vi "仪器电源管理.vi"() -> ()   [LabVIEW 2016, in "环境动力监测库.lvlib" / "V电源管理库.lvlib"]
uses:
  <vilib>/Utility/miscctls.llb/LVPointTypeDef.ctl
  <vilib>/ptbypt/NI_PtbyPt.lvlib
panel:
  out "R115":i16 caption="灯带关闭时间"
  out "R114":i16 caption="灯带开启时间"
  in  "照明":bool
  in  "侧边灯带":bool
  in  "电源控制":T1
  in  "主屏看门狗启用":u16(ring) caption="主屏看门狗启用：" items=["关闭", "打开"]
  in  "主屏看门狗设置":i16 caption="主屏看门狗设置："
  out "主屏看门狗计时":i16 caption="主屏看门狗计时："
  # "仪器电源管理"
  # "H"
  # "H"
  # "s"
  # "s"
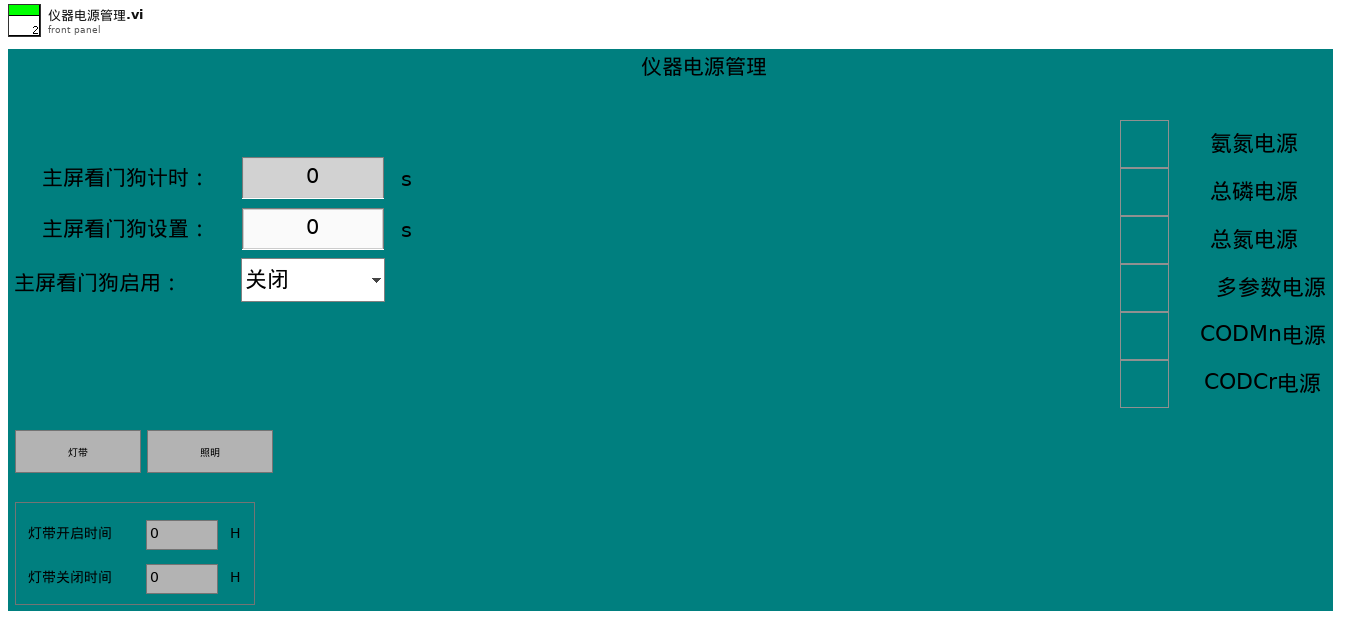
[diagram p1: front panel]
types:
  T1 = cluster{"氨氮电源":bool, "总磷电源":bool, "总氮电源":bool, "多参数电源":bool, "CODMn电源":bool, "CODCr电源":bool}
  T2 = typedef "LVPointTypeDef.ctl" = cluster{"Horizontal":i16, "Vertical":i16}
  T3 = cluster{"状态":cluster{"R0":i16, "R1":i16, "R2":i16, "R3":i16, "R4":i16, "R5":i16, "R6":i16, "R7":i16, "R8":i16, "R9":i16, "R10":i16, "R11":i16, "R12":i16, "R13":i16, "R14":i16, "R15":i16, "R16":i16, "R17":i16, "R18":i16, "R19":i16, "R20":i16, "R21":i16, "R22":i16, "R23":i16, "R24":i16, "R25":i16, "R26":i16, "R27":i16, "R28":i16, "R29":i16, "R30":i16, "R31":i16, "R32":i16, "R33":i16, "R34":i16, "R35":i16, "R36":i16, "R37":i16, "R38":i16, "R39":i16, "R40":i16, "R41":i16, "R42":i16, "R43":i16, "R44":i16, "R45":i16, "R46":i16, "R47":i16, "R48":i16, "R49":i16, "R50":i16, "R51":i16, "R52":i16, "R53":i16, "R54":i16, "R55":i16, "R56":i16, "R57":i16, "R58":i16, "R59":i16, "R60":i16, "R61":i16, "R62":i16, "R63":i16, "R64":i16, "R65":i16, "R66":i16, "R67":i16, "R68":i16, "R69":i16}, "输入状态":bool[], "输出状态":bool[], "报警簇":bool[], "参数设置":cluster{"R100":i16, "R101":i16, "R102":i16, "R103":i16, "R104":i16, "R105":i16, "R106":i16, "R107":i16, "R108":i16, "R109":i16, "R110":i16, "R111":i16, "R112":i16, "R113":i16, "R114":i16, "R115":i16, "R116":i16, "R117":i16, "R118":i16, "R119":i16, "R120":i16, "R121":i16, "R122":i16, "R123":i16, "R124":i16}, "转换值":cluster{"AD0":sgl, "AD1":sgl, "AD2":sgl, "AD3":sgl, "AD4":sgl, "AD5":sgl}, "看门狗启用":bool, "氨氮模块名称":string, "总磷模块名称":string}
  T4 = cluster{"采配水启用":bool, "CODMn启用":bool, "CODcr启用":bool, "氨氮启用":bool, "总磷启用":bool, "质控单元启用":bool, "流量计启用":bool, "电源管理启用":bool, "其他启用":bool, "多参数启用":bool, "超标留样启用":bool, "总氮启用":bool, "运行模式":enum16{"维护模式", "常规模式", "应急模式", "质控模式"}}
  T5 = cluster{"R100":i16, "R101":i16, "R102":i16, "R103":i16, "R104":i16, "R105":i16, "R106":i16, "R107":i16, "R108":i16, "R109":i16, "R110":i16, "R111":i16, "R112":i16, "R113":i16, "R114":i16, "R115":i16, "R116":i16, "R117":i16, "R118":i16, "R119":i16, "R120":i16, "R121":i16, "R122":i16, "R123":i16, "R124":i16}
  T6 = cluster{"R0":i16, "R1":i16, "R2":i16, "R3":i16, "R4":i16, "R5":i16, "R6":i16, "R7":i16, "R8":i16, "R9":i16, "R10":i16, "R11":i16, "R12":i16, "R13":i16, "R14":i16, "R15":i16, "R16":i16, "R17":i16, "R18":i16, "R19":i16, "R20":i16, "R21":i16, "R22":i16, "R23":i16, "R24":i16, "R25":i16, "R26":i16, "R27":i16, "R28":i16, "R29":i16, "R30":i16, "R31":i16, "R32":i16, "R33":i16, "R34":i16, "R35":i16, "R36":i16, "R37":i16, "R38":i16, "R39":i16, "R40":i16, "R41":i16, "R42":i16, "R43":i16, "R44":i16, "R45":i16, "R46":i16, "R47":i16, "R48":i16, "R49":i16, "R50":i16, "R51":i16, "R52":i16, "R53":i16, "R54":i16, "R55":i16, "R56":i16, "R57":i16, "R58":i16, "R59":i16, "R60":i16, "R61":i16, "R62":i16, "R63":i16, "R64":i16, "R65":i16, "R66":i16, "R67":i16, "R68":i16, "R69":i16}
  T7 = cluster{"命令":string, "data":cluster{"starting address":u16, "coil values":bool[]}}
  T8 = cluster{"命令":string, "数据":cluster{"starting address":u16, "holding register values":u16[]}}
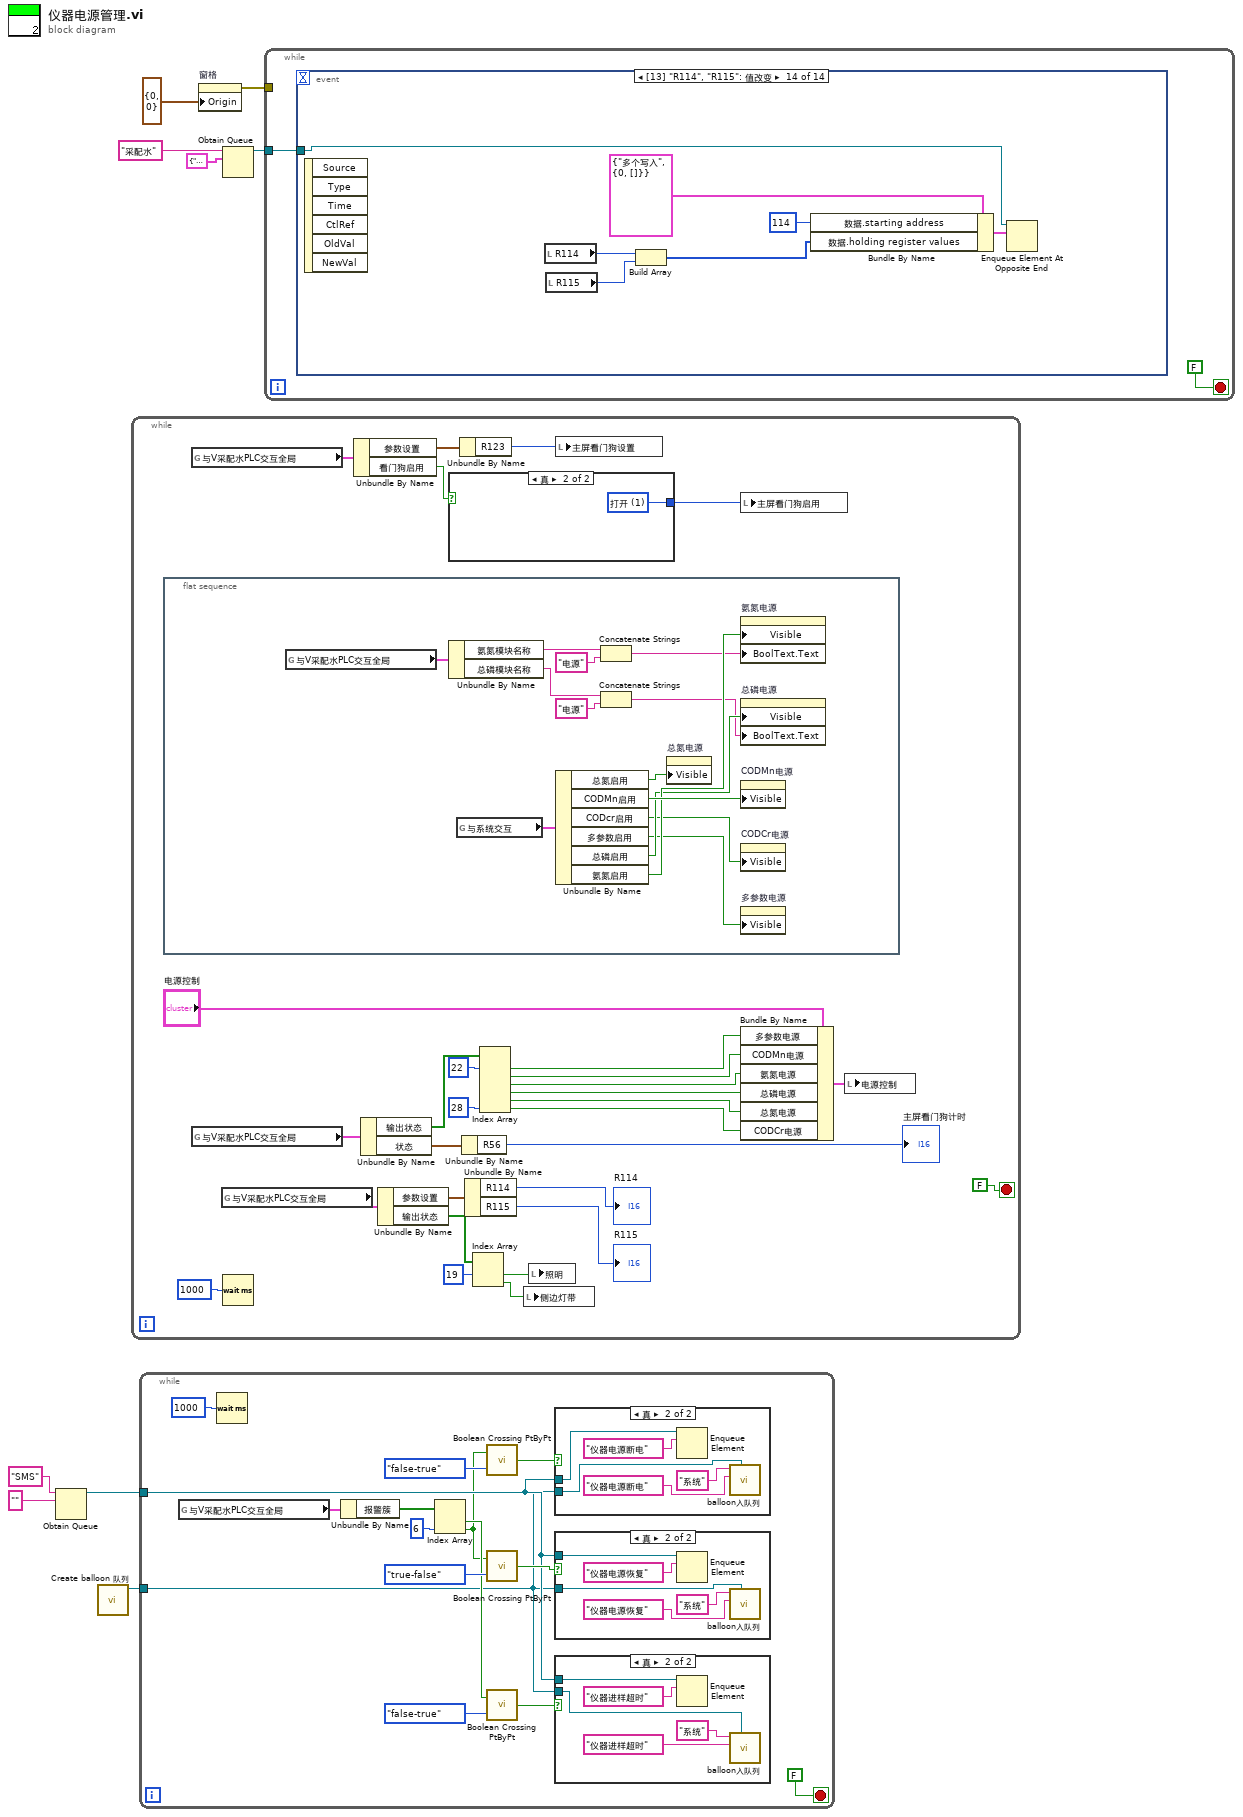
[diagram p0: block diagram]
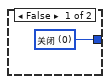
[diagram p5: hidden frame]
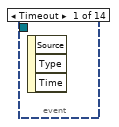
[diagram p6: hidden frame]
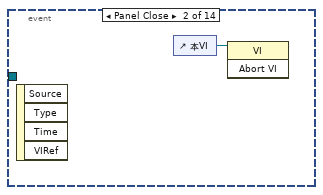
[diagram p7: hidden frame]
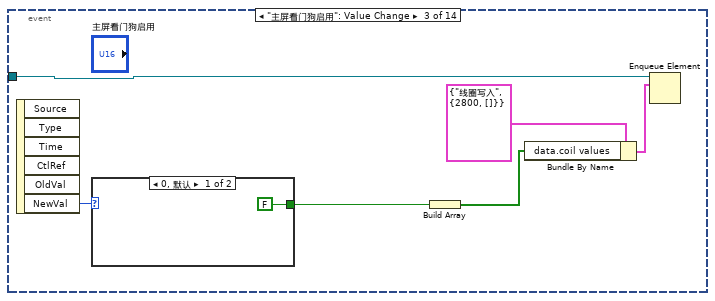
[diagram p8: hidden frame]
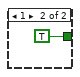
[diagram p9: hidden frame]
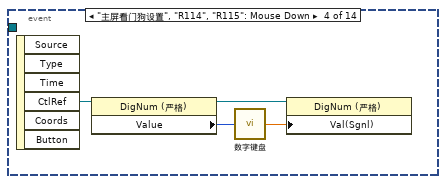
[diagram p10: hidden frame]
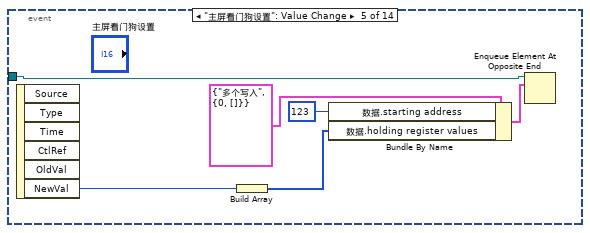
[diagram p11: hidden frame]
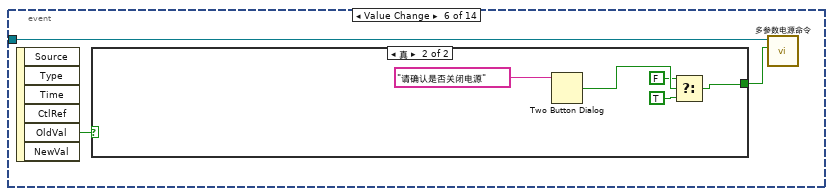
[diagram p12: hidden frame]
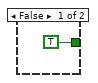
[diagram p13: hidden frame]
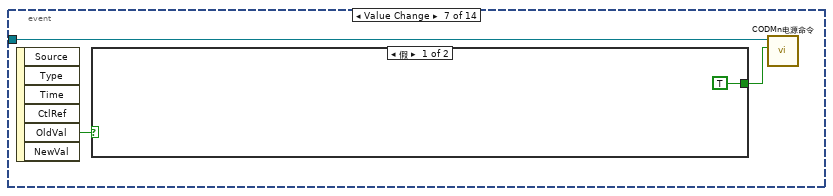
[diagram p14: hidden frame]
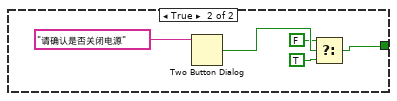
[diagram p15: hidden frame]
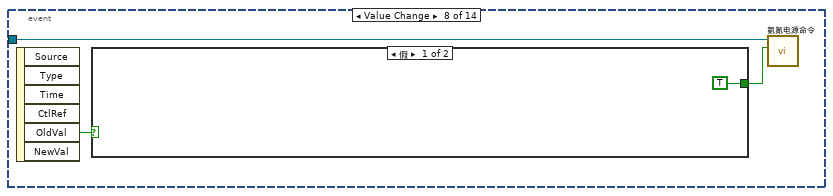
[diagram p16: hidden frame]
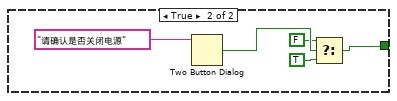
[diagram p17: hidden frame]
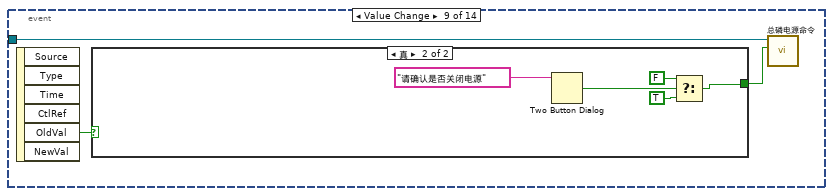
[diagram p18: hidden frame]
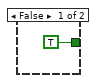
[diagram p19: hidden frame]
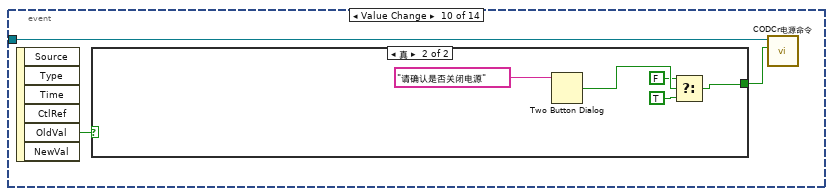
[diagram p20: hidden frame]
diagram:
  n1 = Obtain Queue(name (unnamed)="SMS" ("名称（未命名）"), element data type="" ("名称（未命名）")) -> (queue out=w2:refnum<queue>)  [unwired: 3 in, 2 out]
  n2 = call "Create balloon 队列.vi"() -> ("队列输出"=w1:refnum<queue>)  [unwired: 11 in]
  n3 = while {
    stop <- FALSE stop-if-true
    n4 = flat-sequence {
      frame #0 {
        n5 = global read "外部交互全局变量.vi" "与V采配水PLC交互全局"() -> (w46:T3)
        n6 = Unbundle By Name(w46) -> ("氨氮模块名称"=w45:string, "总磷模块名称"=w42:string)
        n7 = global read "外部交互全局变量.vi" "与系统交互"() -> (w54:T4)
        n8 = Unbundle By Name(w54) -> ("总氮启用"=w53:bool, "CODMn启用"=w52:bool, "CODcr启用"=w48:bool, "多参数启用"=w49:bool, "总磷启用"=w50:bool, "氨氮启用"=w51:bool)
        n9 = Concatenate Strings(w45, "电源" ("字符串")) -> (w44:string)
        n10 = Concatenate Strings(w42, "电源" ("字符串")) -> (w41:string)
        n11 = property on="总氮电源" class="Bool (严格)"("Visible"=w53) -> ()  [unwired: 2 in, 2 out]
        n12 = property on="氨氮电源" class="Bool (严格)"("Visible"=w51, "BoolText.Text"=w44) -> ()  [unwired: 2 in, 2 out]
        n13 = property on="总磷电源" class="Bool (严格)"("Visible"=w50, "BoolText.Text"=w41) -> ()  [unwired: 2 in, 2 out]
        n14 = property on="CODMn电源" class="Bool (严格)"("Visible"=w52) -> ()  [unwired: 2 in, 2 out]
        n15 = property on="CODCr电源" class="Bool (严格)"("Visible"=w48) -> ()  [unwired: 2 in, 2 out]
        n16 = property on="多参数电源" class="Bool (严格)"("Visible"=w49) -> ()  [unwired: 2 in, 2 out]
      }
    }
    n17 = global read "外部交互全局变量.vi" "与V采配水PLC交互全局"() -> (w25:T3)
    n18 = global read "外部交互全局变量.vi" "与V采配水PLC交互全局"() -> (w23:T3)
    n19 = global read "外部交互全局变量.vi" "与V采配水PLC交互全局"() -> (w17:T3)
    n20 = Wait (ms)(milliseconds to wait=u32 1000 ("等待时间（毫秒）")) -> ()  [unwired: 1 out]
    n21 = Unbundle By Name(w25) -> ("参数设置"=w24:T5, "看门狗启用"=w19:bool)
    n22 = Unbundle By Name(w23) -> ("输出状态"=w21:bool[], "状态"=w22:T6)
    n23 = Unbundle By Name(w17) -> ("参数设置"=w16:T5, "输出状态"=w12:bool[])
    n24 = case shown="真" w19 {
      tunnel: [w39 w40] -> w18
      frame False {
        w39 = u16 0 items=["关闭", "打开"] ("主屏看门狗启用")
      }
      frame True {
        w40 = u16 1 items=["关闭", "打开"] ("主屏看门狗启用")
      }
    }
    n25 = Unbundle By Name(w24) -> ("R123"=w35:i16)
    n26 = Unbundle By Name(w22) -> ("R56"=→"主屏看门狗计时":i16)
    n27 = Unbundle By Name(w16) -> ("R114"=→"R114":i16, "R115"=→"R115":i16)
    n28 = Index Array(array=w12, index #1=19 ("索引")) -> (element #1=w11:bool, element #2=w10:bool)  [unwired: 1 in]
    n29 = Index Array(array=w21, index #1=22 ("索引"), index #6=28 ("索引")) -> (element #1=w32:bool, element #2=w31:bool, element #3=w30:bool, element #4=w29:bool, element #5=w28:bool, element #6=w27:bool)  [unwired: 4 in]
    n30 = local write "侧边灯带"(w10) -> ()
    n31 = local write "照明"(w11) -> ()
    n32 = local write "主屏看门狗设置"(w35) -> ()
    n33 = local write "主屏看门狗启用"(w18) -> ()
    n34 = Bundle By Name(cluster="电源控制", "多参数电源"=w32, "CODMn电源"=w31, "氨氮电源"=w30, "总磷电源"=w29, "总氮电源"=w28, "CODCr电源"=w27) -> (w26:T1)
    n35 = local write "电源控制"(w26) -> ()
  }
  n36 = while {
    tunnel: w2 -> [w63]
    tunnel: w1 -> [w57]
    stop <- FALSE stop-if-true
    n37 = global read "外部交互全局变量.vi" "与V采配水PLC交互全局"() -> (w56:T3)
    n38 = Wait (ms)(milliseconds to wait=u32 1000 ("等待时间（毫秒）")) -> ()  [unwired: 1 out]
    n39 = Unbundle By Name(w56) -> ("报警簇"=w55:bool[])
    n40 = Index Array(array=w55, index #2=6 ("索引")) -> (element #1=w60:bool, element #2=w58:bool)  [unwired: 1 in]
    n41 = call <vilib>:"Boolean Crossing PtByPt.vi"("direction"=enum16{"either", "false-true", "true-false"}."false-true", "input"=w58) -> ("crossing"=w66:bool)  [unwired: 1 in]
    n42 = call <vilib>:"Boolean Crossing PtByPt.vi"("direction"=enum16{"either", "false-true", "true-false"}."true-false", "input"=w58) -> ("crossing"=w64:bool)  [unwired: 1 in]
    n43 = call <vilib>:"Boolean Crossing PtByPt.vi"("direction"=enum16{"either", "false-true", "true-false"}."false-true", "input"=w60) -> ("crossing"=w61:bool)  [unwired: 1 in]
    n44 = case shown="真" w66 {
      tunnel: w63 -> [_ w84]
      tunnel: w57 -> [_ w82]
      frame False {
      }
      frame True {
        n45 = Enqueue Element(queue=w84, element="仪器电源断电" ("元素")) -> ()  [unwired: 2 in, 3 out]
        n46 = call "balloon入队列.vi"("队列"=w82, "故障信息"="仪器电源断电" ("元素"), "参数名称"="系统") -> ()  [unwired: 8 in, 1 out]
      }
    }
    n47 = case shown="真" w64 {
      tunnel: w63 -> [_ w77]
      tunnel: w57 -> [_ w76]
      frame False {
      }
      frame True {
        n48 = Enqueue Element(queue=w77, element="仪器电源恢复" ("元素")) -> ()  [unwired: 2 in, 3 out]
        n49 = call "balloon入队列.vi"("队列"=w76, "故障信息"="仪器电源恢复" ("元素"), "参数名称"="系统") -> ()  [unwired: 8 in, 1 out]
      }
    }
    n50 = case shown="真" w61 {
      tunnel: w63 -> [_ w74]
      tunnel: w57 -> [_ w72]
      frame False {
      }
      frame True {
        n51 = Enqueue Element(queue=w74, element="仪器进样超时" ("元素")) -> ()  [unwired: 2 in, 3 out]
        n52 = call "balloon入队列.vi"("队列"=w72, "故障信息"="仪器进样超时" ("元素"), "参数名称"="系统") -> ()  [unwired: 8 in, 1 out]
      }
    }
  }
  n53 = property on="窗格" class="Pane"("Origin"=T2 {"Horizontal"=0, "Vertical"=0} ("原点")) -> (error out=w6:errorcluster)  [unwired: 2 in, 1 out]
  n54 = Obtain Queue(name (unnamed)="采配水" ("名称（未命名）"), element data type=cluster{"命令":string, "数据":variant} {"命令"="", "数据"=variant}) -> (queue out=w5:refnum<queue>)  [unwired: 3 in, 2 out]
  n55 = while {
    tunnel: w5 -> [w86]
    tunnel: w6 -> [_]
    stop <- FALSE stop-if-true
    n56 = event shown="[13] \"R114\", \"R115\": 值改变" {
      selector: _ -> [_ _ _ _ _ _ _ _ _ _ _ _ _ _]
      dyn-events: _ -> [_ _ _ _ _ _ _ _ _ _ _ _ _ _]
      timeout: _ -> [_ _ _ _ _ _ _ _ _ _ _ _ _ _]
      tunnel: w86 -> [_ _ w90 _ w102 w108 w117 w126 w135 w144 w153 w161 w166 w172]
      event Timeout {
        n57 = event-data() -> ()  [unwired: 1 in, 3 out]
      }
      event Panel Close {
        n58 = event-data() -> ()  [unwired: 1 in, 4 out]
        n59 = control-ref of="本VI"() -> (w87:refnum<vi>)
        n60 = invoke class="VI" method="Abort VI"(reference=w87) -> ()  [unwired: 2 in, 3 out]
      }
      event "主屏看门狗启用": Value Change {
        n61 = event-data() -> ("NewVal"=w89:u16)  [unwired: 1 in, 5 out]
        n62 = case shown="0, 默认" w89 {
          tunnel: [FALSE TRUE] -> w88
          frame 0, Default {
          }
          frame 1 {
          }
        }
        n63 = Build Array(w88) -> (w91:bool[])
        n64 = Bundle By Name(cluster=T7 {"命令"="线圈写入", "data"={"starting address"=2800, "coil values"=[]}} ("元素"), "data.coil values"=w91) -> (w92:T7)
        n65 = Enqueue Element(queue=w90, element=w92) -> ()  [unwired: 2 in, 3 out]
      }
      event "主屏看门狗设置", "R114", "R115": Mouse Down {
        n66 = event-data() -> ("CtlRef"=w96:refnum<vi>)  [unwired: 1 in, 5 out]
        n67 = property class="DigNum (严格)"(reference=w96) -> (reference out=w98:refnum<vi>, "Value"=w99:i16)  [unwired: 1 in, 1 out]
        n68 = call "数字键盘.vi"("OldNumber"=w99) -> ("NewNumber"=w97:sgl)
        n69 = property class="DigNum (严格)"(reference=w98, "Val(Sgnl)"=w97) -> ()  [unwired: 1 in, 2 out]
      }
      event "主屏看门狗设置": Value Change {
        n70 = event-data() -> ("NewVal"=w100:i16)  [unwired: 1 in, 5 out]
        n71 = Build Array(w100) -> (w101:i16[])
        n72 = Bundle By Name(cluster=T8 {"命令"="多个写入", "数据"={"starting address"=0, "holding register values"=[]}} ("元素"), "数据.starting address"=u16 123, "数据.holding register values"=w101) -> (w103:T8)
        n73 = Enqueue Element At Opposite End(queue=w102, element=w103) -> ()  [unwired: 2 in, 3 out]
      }
      event "电源控制.多参数电源": Value Change {
        n74 = event-data() -> ("OldVal"=w107:bool)  [unwired: 1 in, 5 out]
        n75 = case shown="真" w107 {
          tunnel: [TRUE ("T button?") w110] -> w106
          frame False {
          }
          frame True {
            n76 = Two Button Dialog(message="请确认是否关闭电源" ("消息")) -> (T button?=w113:bool)  [unwired: 2 in]
            n77 = Select(t=FALSE, s=w113, f=TRUE ("T button?")) -> (s? t:f=w110:bool)
          }
        }
        n78 = call "多参数电源命令.vi"("通电/断电"=w106, "队列"=w108) -> ()  [unwired: 9 in, 1 out]
      }
      event "电源控制.CODMn电源": Value Change {
        n79 = event-data() -> ("OldVal"=w116:bool)  [unwired: 1 in, 5 out]
        n80 = case shown="假" w116 {
          tunnel: [TRUE ("T button?") w119] -> w115
          frame False {
          }
          frame True {
            n81 = Two Button Dialog(message="请确认是否关闭电源" ("消息")) -> (T button?=w122:bool)  [unwired: 2 in]
            n82 = Select(t=FALSE, s=w122, f=TRUE ("T button?")) -> (s? t:f=w119:bool)
          }
        }
        n83 = call "CODMn电源命令.vi"("通电/断电"=w115, "队列"=w117) -> ()  [unwired: 9 in, 1 out]
      }
      event "电源控制.氨氮电源": Value Change {
        n84 = event-data() -> ("OldVal"=w125:bool)  [unwired: 1 in, 5 out]
        n85 = case shown="假" w125 {
          tunnel: [TRUE ("T button?") w128] -> w124
          frame False {
          }
          frame True {
            n86 = Two Button Dialog(message="请确认是否关闭电源" ("消息")) -> (T button?=w131:bool)  [unwired: 2 in]
            n87 = Select(t=FALSE, s=w131, f=TRUE ("T button?")) -> (s? t:f=w128:bool)
          }
        }
        n88 = call "氨氮电源命令.vi"("通电/断电"=w124, "队列"=w126) -> ()  [unwired: 9 in, 1 out]
      }
      event "电源控制.总磷电源": Value Change {
        n89 = event-data() -> ("OldVal"=w134:bool)  [unwired: 1 in, 5 out]
        n90 = case shown="真" w134 {
          tunnel: [TRUE ("T button?") w137] -> w133
          frame False {
          }
          frame True {
            n91 = Two Button Dialog(message="请确认是否关闭电源" ("消息")) -> (T button?=w140:bool)  [unwired: 2 in]
            n92 = Select(t=FALSE, s=w140, f=TRUE ("T button?")) -> (s? t:f=w137:bool)
          }
        }
        n93 = call "总磷电源命令.vi"("通电/断电"=w133, "队列"=w135) -> ()  [unwired: 9 in, 1 out]
      }
      event "电源控制.CODCr电源": Value Change {
        n94 = event-data() -> ("OldVal"=w143:bool)  [unwired: 1 in, 5 out]
        n95 = case shown="真" w143 {
          tunnel: [TRUE ("T button?") w146] -> w142
          frame False {
          }
          frame True {
            n96 = Two Button Dialog(message="请确认是否关闭电源" ("消息")) -> (T button?=w149:bool)  [unwired: 2 in]
            n97 = Select(t=FALSE, s=w149, f=TRUE ("T button?")) -> (s? t:f=w146:bool)
          }
        }
        n98 = call "CODCr电源命令.vi"("通电/断电"=w142, "队列"=w144) -> ()  [unwired: 9 in, 1 out]
      }
      event "电源控制.总氮电源": Value Change {
        n99 = event-data() -> ("OldVal"=w151:bool)  [unwired: 1 in, 5 out]
        n100 = case shown="真" w151 {
          tunnel: [TRUE ("T button?") w155] -> w152
          frame False {
          }
          frame True {
            n101 = Two Button Dialog(message="请确认是否关闭电源" ("消息")) -> (T button?=w158:bool)  [unwired: 2 in]
            n102 = Select(t=FALSE, s=w158, f=TRUE ("T button?")) -> (s? t:f=w155:bool)
          }
        }
        n103 = call "总氮电源命令.vi"("通电/断电"=w152, "队列"=w153) -> ()  [unwired: 9 in, 1 out]
      }
      event "侧边灯带": Value Change {
        n104 = event-data() -> ()  [unwired: 1 in, 6 out]
        n105 = Build Array("侧边灯带") -> (w162:bool[])
        n106 = Bundle By Name(cluster=T7 {"命令"="线圈写入", "data"={"starting address"=2450, "coil values"=[]}} ("元素"), "data.coil values"=w162) -> (w163:T7)
        n107 = Enqueue Element(queue=w161, element=w163) -> ()  [unwired: 2 in, 3 out]
      }
      event "照明": Value Change {
        n108 = event-data() -> ()  [unwired: 1 in, 6 out]
        n109 = Build Array("照明") -> (w167:bool[])
        n110 = Bundle By Name(cluster=T7 {"命令"="线圈写入", "data"={"starting address"=2452, "coil values"=[]}} ("元素"), "data.coil values"=w167) -> (w168:T7)
        n111 = Enqueue Element(queue=w166, element=w168) -> ()  [unwired: 2 in, 3 out]
      }
      event "R114", "R115": Value Change {
        n112 = event-data() -> ()  [unwired: 1 in, 6 out]
        n113 = local read "R114"() -> (w171:i16)
        n114 = local read "R115"() -> (w170:i16)
        n115 = Build Array(w171, w170) -> (w173:i16[])
        n116 = Bundle By Name(cluster=T8 {"命令"="多个写入", "数据"={"starting address"=0, "holding register values"=[]}} ("元素"), "数据.starting address"=u16 114, "数据.holding register values"=w173) -> (w174:T8)
        n117 = Enqueue Element At Opposite End(queue=w172, element=w174) -> ()  [unwired: 2 in, 3 out]
      }
    }
  }
